vi "sub_calcpadding-symbolrate.vi"(2 "Tx IQ Sampling\nRate [s/sec]":dbl, 3 "Samples per Symbol":i32) -> (0 "Symbol Rate":dbl, 1 "Padding Bits":i32)   [LabVIEW 2012]
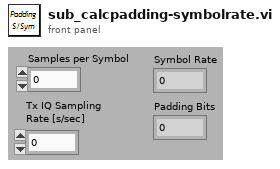
[diagram p1: front panel]
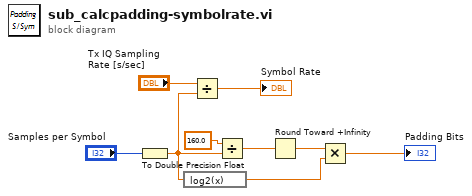
[diagram p0: block diagram]
diagram:
  n1 = To Double Precision Float(number="Samples per Symbol") -> (double precision float=w8:dbl)
  n2 = expression code="log2(x)"(w8) -> (w5:dbl)
  n3 = Divide(x="Tx IQ Sampling\nRate [s/sec]", y=w8) -> (x/y=→"Symbol Rate":dbl)
  n4 = Divide(x=160.0, y=w8) -> (x/y=w3:dbl)
  n5 = Round Toward +Infinity(x=w3) -> (ceil(x): smallest int >= x=w4:dbl)
  n6 = Multiply(x=w4, y=w5) -> (x*y=→"Padding Bits":dbl)
